vi "ifft_peaks.vi"() -> ()   [LabVIEW 2009]
uses:
  <vilib>/Analysis/2dsp.llb/Inverse Real FFT.vi
  <vilib>/Analysis/NI_AALPro.lvlib
panel:
  out "Waveform Graph":dbl[](graph)
  in  "resolution d(Hz)":dbl(slide) scale=0.0..1.0
  out "X":dbl[](array[numeric])
  in  "fundamental frequency":dbl(slide) scale=0.0..3.0
  in  "peaks":dbl[](array[numeric])
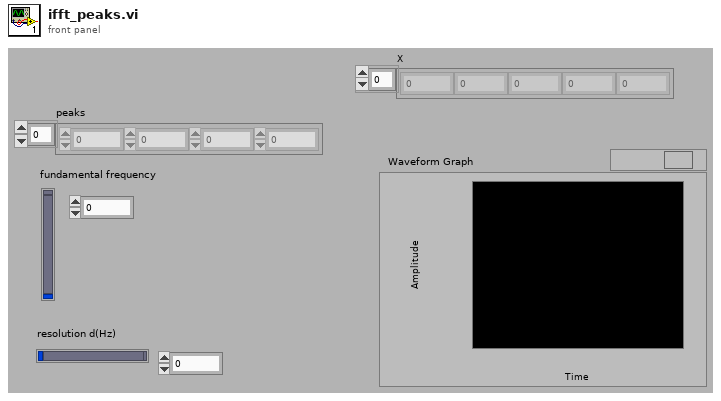
[diagram p1: front panel]
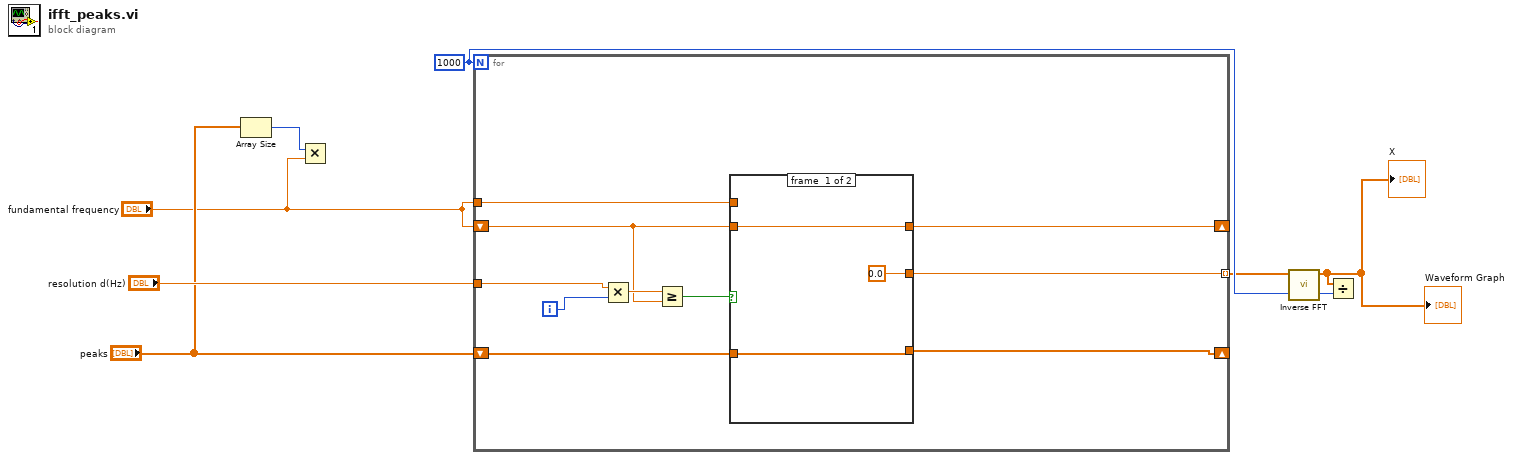
[diagram p0: block diagram]
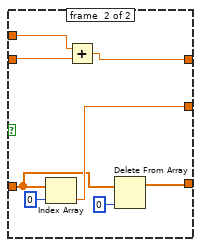
[diagram p2: hidden frame]
diagram:
  w3 = 1000
  n1 = Array Size(array="peaks") -> (size(s)=w5:i32)
  n2 = Multiply(x=w5, y="fundamental frequency") -> ()  [unwired: 1 out]
  n3 = for {
    N: w3 -> [_]
    shift-right: [w9] -> _
    shift-left: "peaks" -> [w10]
    tunnel: "fundamental frequency" -> [w13]
    shift-right: [w12] -> _
    shift-left: "fundamental frequency" -> [w14]
    tunnel: [w11] -> w2 mode=indexing
    tunnel: "resolution d(Hz)" -> [w8]
    i -> [w17]
    n4 = Multiply(x=w8, y=w17) -> (x*y=w16:dbl)
    n5 = Greater Or Equal?(x=w16, y=w14) -> (x >= y?=w15:bool)
    n6 = case shown="True" w15 {
      tunnel: w14 -> [w20 w28]
      tunnel: w13 -> [_ w27]
      tunnel: [w20 w26] -> w12
      tunnel: [0.0 w24] -> w11
      tunnel: w10 -> [w18 w23]
      tunnel: [w18 w21] -> w9
      frame #0 {
      }
      frame #1 {
        n7 = Index Array(array=w23, index=0) -> (element=w24:dbl)
        n8 = Add(x=w27, y=w28) -> (x+y=w26:dbl)
        n9 = Delete From Array(array=w23, index=0) -> (array with subset deleted=w21:dbl[])  [unwired: 1 in, 1 out]
      }
    }
  }
  n10 = call-poly <vilib>:"Inverse FFT.vi"("FFT {X}"=w2) -> ("X"=w1:dbl[])  [unwired: 1 in, 9 out]
  "X" <- w1
  "Waveform Graph" <- w1
  n11 = Divide(x=w1, y=w3) -> ()  [unwired: 1 out]
